vi "Eval Single-Variable Array.vi"(2 "error in (no error)":errorcluster, 3 "X Values":dbl[](array[numeric]) format="%0.2f", 4 "formula":string) -> (0 "error out":errorcluster, 1 "Y Values":dbl[](array[numeric]) format="%0.2f")   [LabVIEW 2017, in "NI_Gmath.lvlib"]
doc: "Calculates an array of function values at given points in a given interval by y[i] = f(x[i]) for i = 1, ...n, where f is the 1D function given by the user formula."
uses:
  <vilib>/gmath/NI_Gmath.lvlib
panel:
  # "Example:\n\n formula: x*sin(x)\n X Values: (1.0,1.56,3.14)"
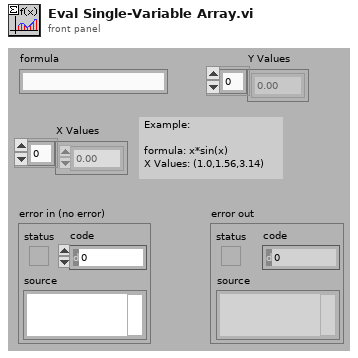
[diagram p1: front panel]
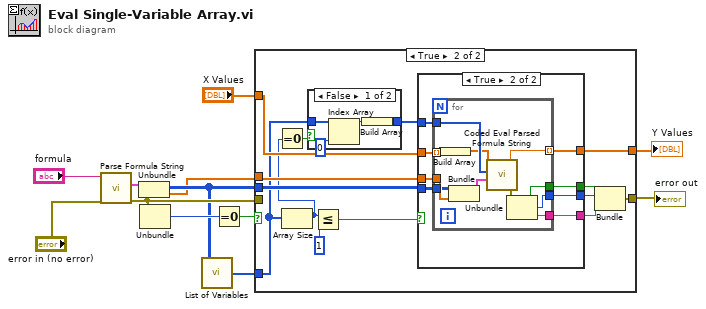
[diagram p0: block diagram]
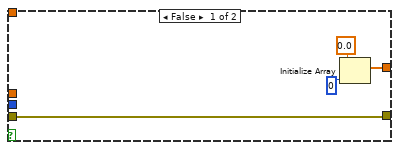
[diagram p2: hidden frame]
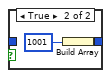
[diagram p3: hidden frame]
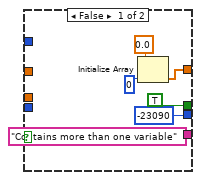
[diagram p4: hidden frame]
diagram:
  n1 = call <vilib>:"Parse Formula String.vi"("error in (no error)"="error in (no error)", "formula"="formula") -> ("error out"=w8:errorcluster, "Parsed Formula"=w5:cluster{"Table":i32[][], "Y Values":dbl[]})
  n2 = Unbundle(w5) -> ("Table"=w4:i32[][], "Y Values"=w3:dbl[])
  n3 = Unbundle(w8) -> ("code"=w6:i32)  [unwired: 2 out]
  n4 = call <vilib>:"List of Variables.vi"("Table"=w4) -> ("List of variables"=w11:i32[])
  n5 = Equal To 0?(x=w6) -> (x = 0?=w12:bool)
  n6 = case shown="True" w12 {
    tunnel: [w13 w29] -> w10
    tunnel: w8 -> [w16 _]
    tunnel: w3 -> [_ w28]
    tunnel: w4 -> [_ w30]
    tunnel: w11 -> [_ w24]
    tunnel: "X Values" -> [_ w25]
    tunnel: [w16 w17] -> w1
    frame False {
      n7 = Initialize Array(0.0, 0) -> (w13:dbl[])
    }
    frame True {
      n8 = Array Size(array=w24) -> (size(s)=w22:i32)
      n9 = Equal To 0?(x=w22) -> (x = 0?=w21:bool)
      n10 = case shown="False" w21 {
        tunnel: [w32 w36] -> w23
        tunnel: w24 -> [w31 _]
        frame False {
          n11 = Index Array(array=w31, index=0) -> (element=w33:i32)
          n12 = Build Array(w33) -> (w32:i32[])
        }
        frame True {
          n13 = Build Array(1001) -> (w36:i32[])
        }
      }
      n14 = Less Or Equal?(x=w22, y=1) -> (x <= y?=w26:bool)
      n15 = case shown="True" w26 {
        tunnel: w25 -> [_ w50]
        tunnel: [w37 w49] -> w29
        tunnel: w30 -> [_ w48]
        tunnel: w28 -> [_ w47]
        tunnel: w23 -> [_ w46]
        tunnel: [TRUE w45] -> w20
        tunnel: [-23090 w44] -> w19
        tunnel: ["Contains more than one variable" w43] -> w18
        frame False {
          n16 = Initialize Array(0.0, 0) -> (w37:dbl[])
        }
        frame True {
          n17 = for {
            tunnel: w46 -> [w52]
            tunnel: w47 -> [w55]
            tunnel: w48 -> [w54]
            tunnel: [w61] -> w49 mode=indexing
            tunnel: w50 -> [w60] mode=indexing
            tunnel: [w58] -> w45
            tunnel: [w57] -> w44
            tunnel: [w56] -> w43
            n18 = Build Array(w60) -> (w51:dbl[])
            n19 = Bundle("Table"=w54, "Y Values"=w55) -> (w53:cluster{"Table":i32[][], "Y Values":dbl[]})  [unwired: 1 in]
            n20 = call <vilib>:"Coded Eval Parsed Formula String.vi"("Parsed Formula"=w53, "Variables"=w52, "X Values"=w51) -> ("error out"=w59:errorcluster, "y value"=w61:dbl)  [unwired: 1 in]
            n21 = Unbundle(w59) -> ("status"=w58:bool, "code"=w57:i32, "source"=w56:string)
          }
        }
      }
      n22 = Bundle("status"=w20, "code"=w19, "source"=w18) -> (w17:errorcluster)  [unwired: 1 in]
    }
  }
  "Y Values" <- w10
  "error out" <- w1
